vi "Launch Core Instance.vi"(8 "error in (no error)":errorcluster, 10 "Trigger":bool, 11 "CaptureDetectionLoopDataIn":T1={"Period"=-1, "Reset"=TRUE, "Trigger"=FALSE, "Iteration"=0, "Capture"=path "", "Mode"=enum."Record", "Replay Run ID"="", "Module Launched Timestamp"=timestamp(0 s since 1904-01-01)}) -> (0 "error out":errorcluster, 3 "CaptureDetectionLoopDataOut":T1={"Period"=-1, "Reset"=TRUE, "Trigger"=FALSE, "Iteration"=0, "Capture"=path "", "Mode"=enum."Record", "Replay Run ID"="", "Module Launched Timestamp"=timestamp(0 s since 1904-01-01)})   [LabVIEW 2026, in "Launcher.lvlib"]
uses:
  Launcher.lvlib
  Capture detection loop data--cluster.ctl
  Mode.ctl
  Core/Core.lvlib
  067b5d79-57af-4187-b312-f72a8a32ce84.vi
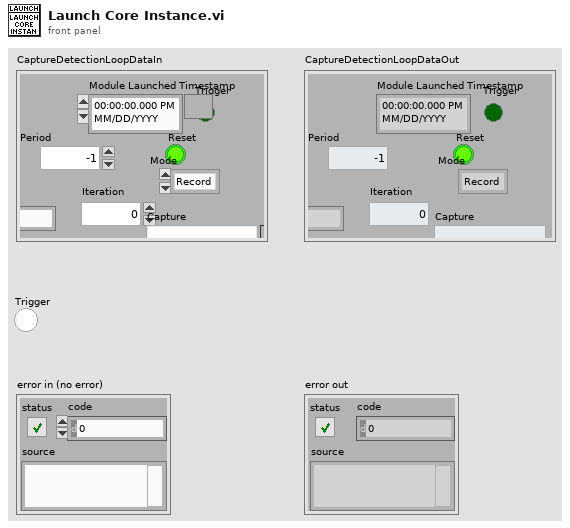
[diagram p1: front panel]
types:
  T1 = typedef "Capture detection loop data--cluster.ctl" = cluster{"Period":i32, "Reset":bool, "Trigger":bool, "Iteration":i32, "Capture":path, "Mode":T2, "Replay Run ID":string, "Module Launched Timestamp":timestamp}
  T2 = typedef "Mode.ctl" = enum16{"Record", "Record and Replay"}
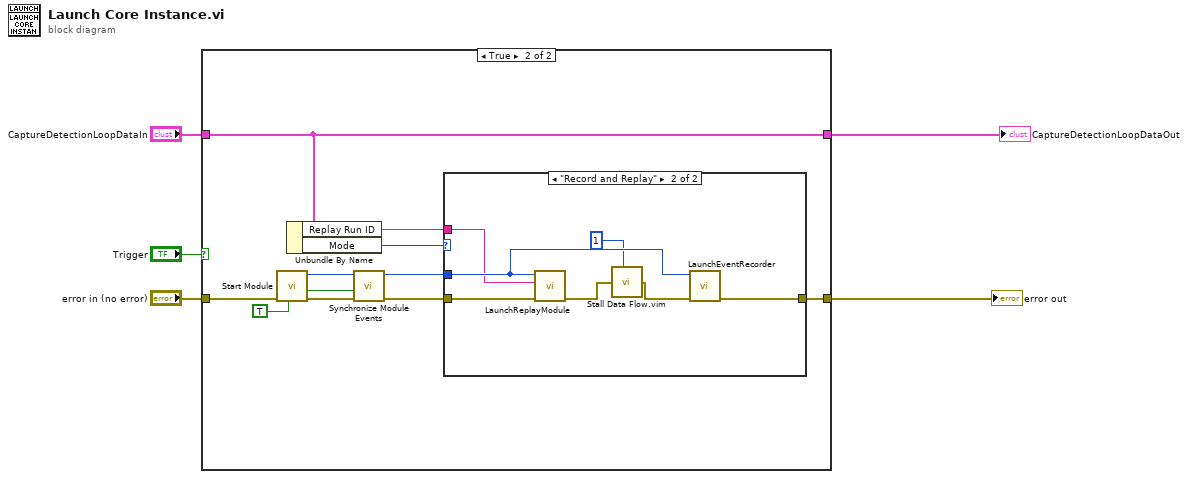
[diagram p0: block diagram]
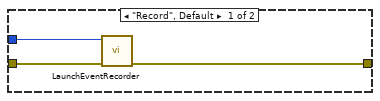
[diagram p3: hidden frame]
diagram:
  n1 = case shown="True" "Trigger" {
    tunnel: "error in (no error)" -> [w6 w16]
    tunnel: [w6 w11] -> w4
    tunnel: "CaptureDetectionLoopDataIn" -> [w7 w10]
    tunnel: [w7 w10] -> w1
    frame False {
    }
    frame True {
      n2 = call "Start Module.vi"("Show Main VI Diagram on Init (F)"=TRUE, "error in"=w16) -> ("error out"=w15:errorcluster, "Wait for Event Sync?"=w18:bool, "Module ID"=w17:i32)  [unwired: 5 in, 2 out]
      n3 = Unbundle By Name(w10) -> ("Replay Run ID"=w8:string, "Mode"=w9:T2)
      n4 = call "Synchronize Module Events.vi"("error in"=w15, "Wait for Event Sync?"=w18, "Module ID in"=w17) -> ("error out"=w13:errorcluster, "Module ID out"=w12:i32)  [unwired: 7 in]
      n5 = case shown="\"Record and Replay\"" w9 {
        tunnel: w13 -> [w21 w28]
        tunnel: w12 -> [w20 w27]
        tunnel: [w19 w26] -> w11
        tunnel: w8 -> [_ w25]
        frame "Record", Default {
          n6 = call "LaunchEventRecorder.vi"("error in"=w21, "Module ID"=w20) -> ("error out"=w19:errorcluster)  [unwired: 9 in]
        }
        frame "Record and Replay" {
          n7 = call "LaunchReplayModule.vi"("error in"=w28, "Run ID"=w25, "Module ID"=w27) -> ("error out"=w24:errorcluster)  [unwired: 8 in]
          n8 = call "Stall Data Flow.vim"("value in"=w24, "milliseconds to wait"=u32 1) -> ("value out"=w23:errorcluster)  [unwired: 1 out]
          n9 = call "LaunchEventRecorder.vi"("error in"=w23, "Module ID"=w27) -> ("error out"=w26:errorcluster)  [unwired: 9 in]
        }
      }
    }
  }
  "CaptureDetectionLoopDataOut" <- w1
  "error out" <- w4
